vi "Ctor.vi"(8 "error in (no error)":errorcluster) -> (0 "error out":errorcluster, 3 "App Watcher out":refnum<class "App Watcher.lvclass">)   [LabVIEW 2020, in "PicoG-App.lvlib" / "App Watcher.lvclass"]
uses:
  App Watcher.lvclass
  ViaApp/ViaApp.lvclass
  App Update Data.ctl
  Ref Data.ctl
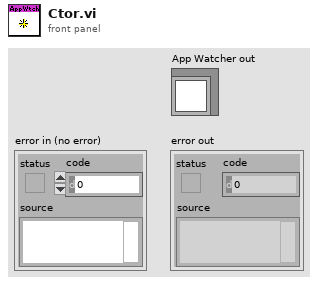
[diagram p1: front panel]
types:
  T1 = typedef "PicoG-App.lvlib/App Watcher.lvclass/Ref Data.ctl" = cluster{"App Map":map{path, refnum<class "ViaApp.lvclass">}, "App Update Event":refnum<user-event>}
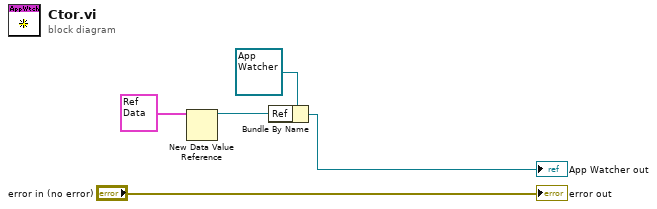
[diagram p0: block diagram]
diagram:
  n1 = New Data Value Reference(data value=T1 {"App Map"={}, "App Update Event"=refnum} ("Ref Data")) -> (data value reference=w1:refnum<data-value>)  [unwired: 1 in, 1 out]
  n2 = Bundle By Name(cluster=refnum<class "App Watcher.lvclass"> refnum ("App Watcher in"), "Ref"=w1) -> (→"App Watcher out":refnum<class "App Watcher.lvclass">)
  "error out" <- "error in (no error)"
